vi "adc_cdc_usb.vi"(0 "VISA resource name":refnum<visa-resource-name>="COM1", 1 "baud rate":u32=9600, 2 "data bits":u16=8 min=5 max=8 step=1, 3 "parity":u16(ring) items=["None", "Odd", "Even", "Mark", "Space"], 4 "stop bits":u16(ring)=10 items=["1.0"=10, "1.5"=15, "2.0"=20], 7 "flow control":u16(ring) items=["None"=0, "XON/XOFF"=1, "RTS/CTS"=2, "DTR/DSR"=4]) -> ()   [LabVIEW 2010]
doc: "The Basic Serial Read and Write example performs a Serial Port Read, a Serial Port Write, or a combination of these actions. The user selects the actions (read or write) on the front panel. If both are selected, the VI will write the data first, read data, and then close the VISA session that is opened to the port. This VI will wait until the specified number of bytes is received at the port. Only the number of bytes specified will be read.\n\nINSTRUCTIONS:\n1) Select the serial resource and configuration parameters (baud rate, data bits, parity, stop bits, flow control).\n2) Select the operations to be performed. \n3) Connect the serial port to your device. If no device is available, perform a loopback test by doing one of the following. Short pins 2 and 3 on a RS-232 cable or short pin 4 to pin 8 and pin 5 to pin 9 on a RS-485/422 cable. \n4) Run the VI to see the data read. (The \"read string\" will match the \"string to write\" if a loopback test was performed.)\n\nNote: The parameters set for the serial port must match the parameters of the connected instrument or device. In this example, the bytes to read parameter specifies the number of bytes that the serial port reads. If there were more bytes at the port than the number specified in bytes to read, those bytes would not be read. Also, if you specify to read more bytes than the number of bytes actually read, you might receive a timeout error message.\n\nOn the block diagram, the Configure Serial Port VI sets the configuration parameters. The front panel displays the controls used to configure the basic parameters, such as baud rate, data bits, and parity. Constants configure the other parameters the user probably does not need set. After the VISA Configure Serial Port VI opens the VISA session and configures the port, the VI passes the VISA resource name to other VIs that perform operations on that VISA resource. The VISA Write function sends a command to the serial device and the VISA Read function returns data based on the command. The VISA Close function then closes the reference to the serial device. It is important to close the reference; otherwise communication through with that port through protocols other than VISA might not be possible."
uses:
  <vilib>/Instr/_visa.llb/VISA Configure Serial Port (Instr).vi
panel:
  out "ESTADO PUSH BUTON":bool
  out "Thermometer":dbl(slide) scale=0.0..500.0
  in  "stop":bool
  in  "LEER PUSH BUTON":bool
  in  "LEER TEMPERATURA":bool
  in  "LED":bool
  in  "BUZZER":bool
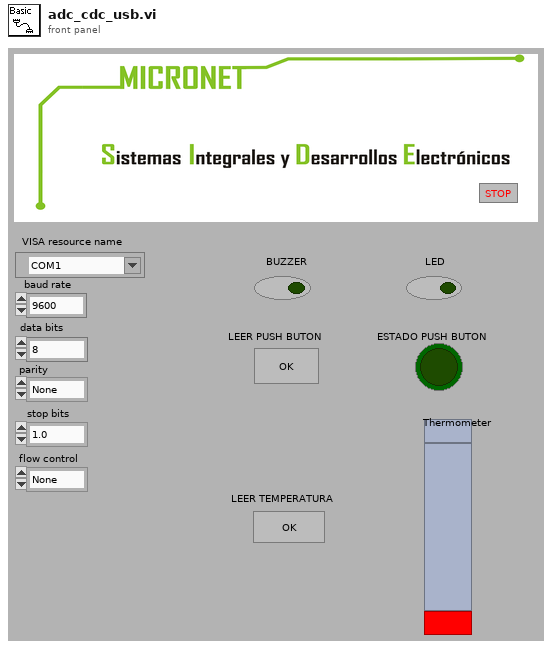
[diagram p1: front panel]
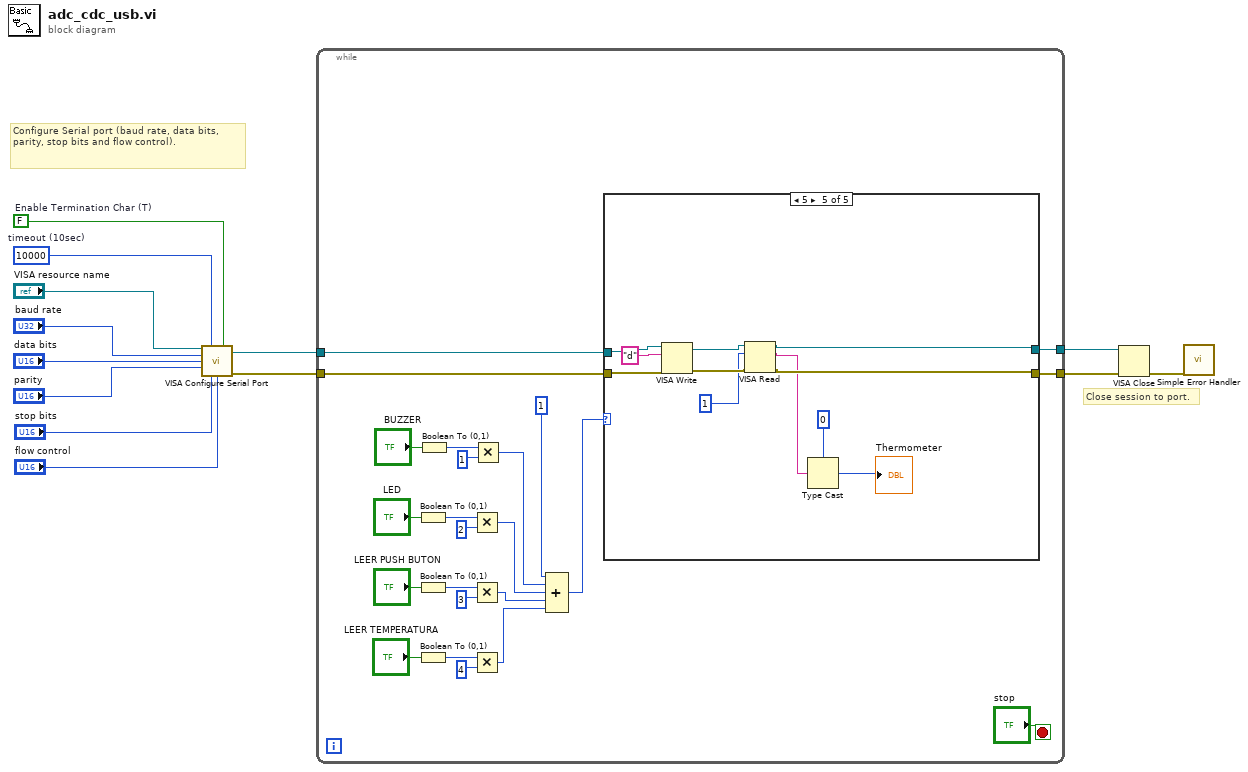
[diagram p0: block diagram]
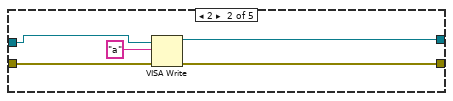
[diagram p3: hidden frame]
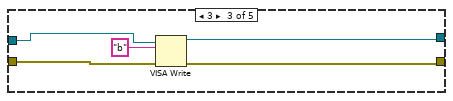
[diagram p4: hidden frame]
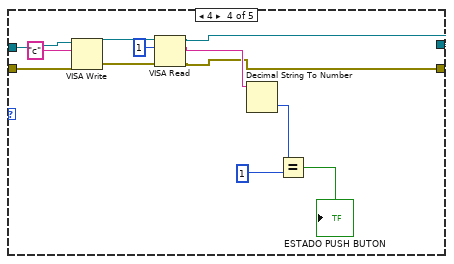
[diagram p5: hidden frame]
diagram:
  w8 = FALSE  # Enable Termination Char (T)
  w9 = u32 10000  # timeout (10sec)
  # "Configure Serial port (baud rate, data bits, parity, stop bits and flow control)."
  # "Close session to port."
  n1 = call-poly "VISA Configure Serial Port"("VISA resource name"="VISA resource name", "timeout (10sec)"=w9, "Enable Termination\nChar (T)"=w8, "baud rate (9600)"="baud rate", "data bits (8)"="data bits", "parity (0:none)"="parity", "stop bits (10: 1 bit)"="stop bits", "flow control (0:none)"="flow control") -> ("VISA resource name out"=w4:refnum<visa-resource-name>, "error out"=w3:errorcluster)  [unwired: 1 in, 5 out]
  n2 = while {
    tunnel: w4 -> [w22]
    tunnel: w3 -> [w21]
    tunnel: [w20] -> w2
    tunnel: [w19] -> w1
    stop <- "stop" stop-if-true
    n3 = Boolean To (0,1)(Boolean="LED") -> (0, 1=w34:i16)
    n4 = Boolean To (0,1)(Boolean="LEER PUSH BUTON") -> (0, 1=w33:i16)
    n5 = Boolean To (0,1)(Boolean="LEER TEMPERATURA") -> (0, 1=w25:i16)
    n6 = Boolean To (0,1)(Boolean="BUZZER") -> (0, 1=w35:i16)
    n7 = Multiply(x=w34, y=i16 2) -> (x*y=w29:i16)
    n8 = Multiply(x=w33, y=i16 3) -> (x*y=w28:i16)
    n9 = Multiply(x=w25, y=4) -> (x*y=w23:i32)
    n10 = Multiply(x=w35, y=1) -> (x*y=w16:i32)
    n11 = Compound Arithmetic op=ADD(1, w16, w29, w28, w23) -> (w36:i32)
    n12 = case shown="5" w36 {
      tunnel: w22 -> [w37 w42 w47 w59 w69]
      tunnel: w21 -> [w38 w41 w46 w58 w70]
      tunnel: [w37 w40 w45 w54 w66] -> w20
      tunnel: [w38 w39 w44 w52 w65] -> w19
      frame 1, Default {
      }
      frame 2 {
        n13 = VISA Write(VISA resource name=w42, write buffer="a" ("string to write 2"), error in (no error)=w41) -> (VISA resource name out=w40:refnum<visa-resource-name>, error out=w39:errorcluster)  [unwired: 1 out]
      }
      frame 3 {
        n14 = VISA Write(VISA resource name=w47, write buffer="b" ("string to write 2"), error in (no error)=w46) -> (VISA resource name out=w45:refnum<visa-resource-name>, error out=w44:errorcluster)  [unwired: 1 out]
      }
      frame 4 {
        n15 = VISA Write(VISA resource name=w59, write buffer="c" ("string to write 2"), error in (no error)=w58) -> (VISA resource name out=w50:refnum<visa-resource-name>, error out=w51:errorcluster)  [unwired: 1 out]
        n16 = VISA Read(VISA resource name=w50, byte count=u32 1, error in (no error)=w51) -> (VISA resource name out=w54:refnum<visa-resource-name>, read buffer=w53:string, error out=w52:errorcluster)  [unwired: 1 out]
        n17 = Decimal String To Number(string=w53) -> (number=w56:i32)  [unwired: 2 in, 1 out]
        n18 = Equal?(x=w56, y=1) -> (x = y?=→"ESTADO PUSH BUTON":bool)
      }
      frame 5 {
        n19 = VISA Write(VISA resource name=w69, write buffer="d" ("string to write 2"), error in (no error)=w70) -> (VISA resource name out=w63:refnum<visa-resource-name>, error out=w62:errorcluster)  [unwired: 1 out]
        n20 = VISA Read(VISA resource name=w63, byte count=u32 1 ("Bytes to Read"), error in (no error)=w62) -> (VISA resource name out=w66:refnum<visa-resource-name>, read buffer=w64:string, error out=w65:errorcluster)  [unwired: 1 out]
        n21 = Type Cast(type=u8 0, x=w64) -> (*(type *) &x=→"Thermometer":u8)
      }
    }
  }
  n22 = VISA Close(VISA resource name=w2, error in (no error)=w1) -> (error out=w11:errorcluster)
  n23 = call <vilib>:"Simple Error Handler.vi"("error in (no error)"=w11) -> ()  [unwired: 1 in, 8 out]
